vi "Get.vi"(8 "error in":errorcluster, 10 "Sub Index":u8, 11 "Sub Objects Dictionary in":refnum<class "Sub Objects Dictionary.lvclass">) -> (0 "error out":errorcluster, 1 "Sub Obj":refnum<class "Sub Object.lvclass">, 3 "Sub Objects Dictionary out":refnum<class "Sub Objects Dictionary.lvclass">)   [LabVIEW 2020, in "CANopen.lvlib" / "Sub Objects Dictionary.lvclass"]
doc: "Gets the Sub Object associated with the specified index."
uses:
  Sub Objects Dictionary.lvclass
  Sub Objects Dictionary.lvclass/Sub Objects Dictionary.ctl
  Sub Object/Sub Object.lvclass
  Ordered-Dictionary/Ordered Object Dictionary/Source/Ordered Object Dictionary.lvclass
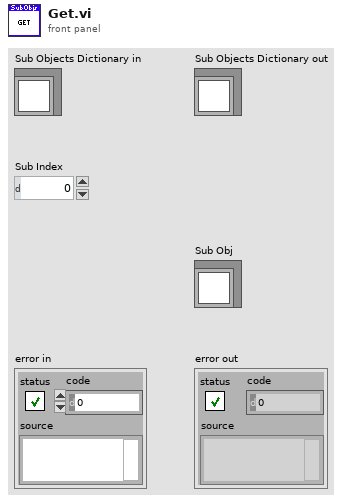
[diagram p1: front panel]
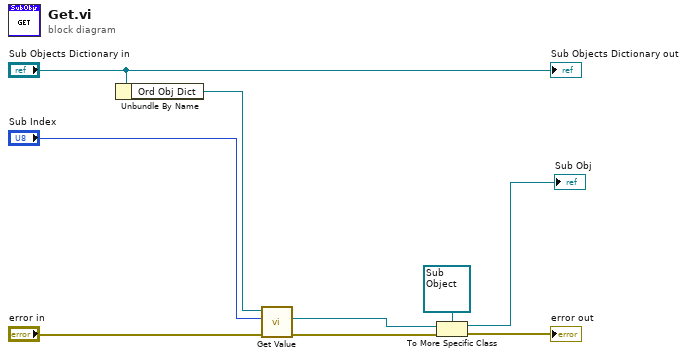
[diagram p0: block diagram]
diagram:
  n1 = Unbundle By Name("Sub Objects Dictionary in") -> ("Ord Obj Dict"=w8:refnum<class "Ordered Object Dictionary.lvclass">)
  n2 = call "Get Value.vi"("error in"="error in", "Key"="Sub Index", "Ordered Object Dictionary in"=w8) -> ("error out"=w6:errorcluster, "Value"=w5:refnum<class>)  [unwired: 6 in, 1 out]
  n3 = To More Specific Class(target class=refnum<class "Sub Object.lvclass"> refnum ("CANopen.lvlib:Sub Obj"), reference=w5, error in=w6) -> (specific class reference=→"Sub Obj":refnum<class "Sub Object.lvclass">, error out=→"error out":errorcluster)
  "Sub Objects Dictionary out" <- "Sub Objects Dictionary in"
